vi "Get Property Value.vi"(8 "error in":errorcluster, 10 "Property Type":T1, 11 "Property Type Node":refnum<k20>) -> (0 "error out":errorcluster, 2 "Property Value":variant, 3 "Property Type Node":refnum<k20>)   [LabVIEW 2024, in "Config File Parser.lvlib" / "Property.lvclass"]
uses:
  Property.lvclass
  Property.lvclass/Property.ctl
  <resource>/objmgr/DOMUserDefRef.rc
  <vilib>/xml/NI_XML.lvlib
  Config File Parser.lvlib
  DependentFile.ctl
  <vilib>/xml/Close Reference(Node).vi
  Property Type.ctl
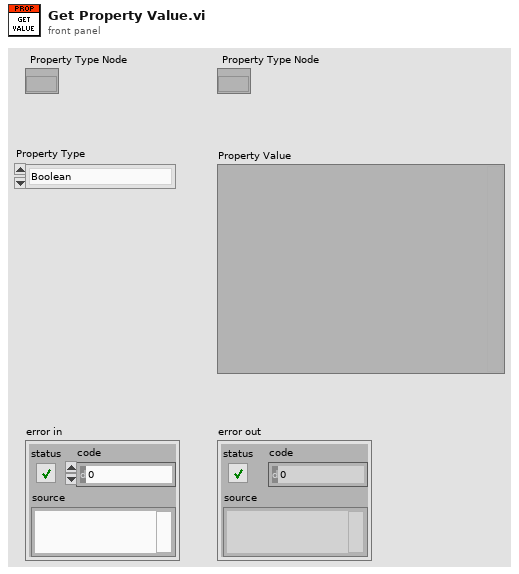
[diagram p1: front panel]
types:
  T1 = typedef "Config File Parser.lvlib/Property.lvclass/Property Type.ctl" = enum16{"Boolean", "Double", "String", "Path", "Dictionary", "DependentFile", "I16", "I32", "I64", "U16", "U32", "U64", "BooleanArray", "DoubleArray", "StringArray", "I16Array", "I32Array", "I64Array", "U16Array", "U32Array", "U64Array"}
  T2 = typedef "Config File Parser.lvlib/Property.lvclass/DependentFile.ctl" = cluster{"Path":string, "Version":string, "RTDestination":string, "ForceDownload":string, "SupportedTarget":string, "MD5":string, " Type":string}
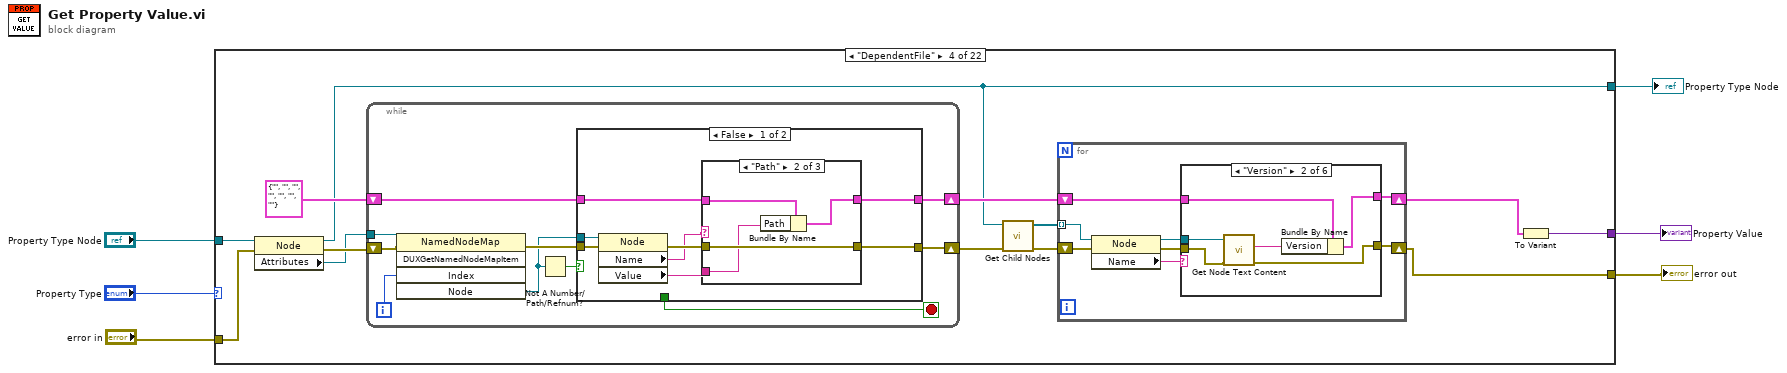
[diagram p0: block diagram]
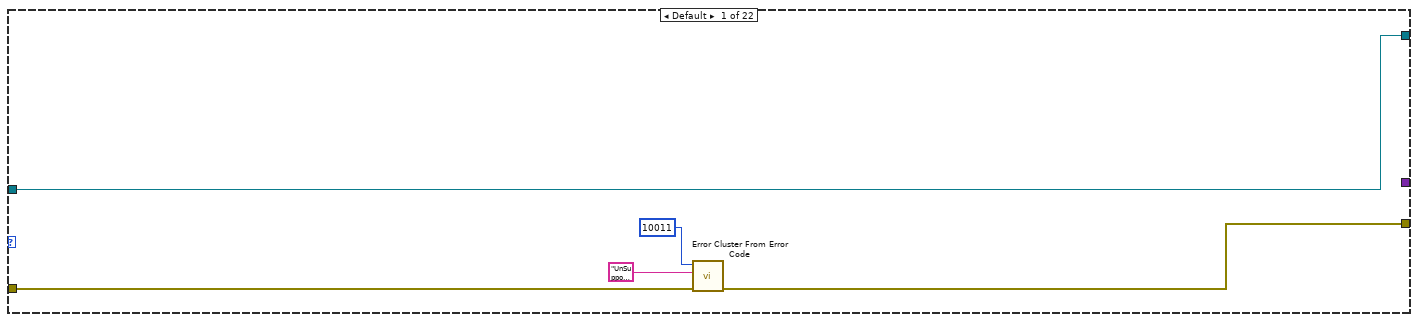
[diagram p2: hidden frame]
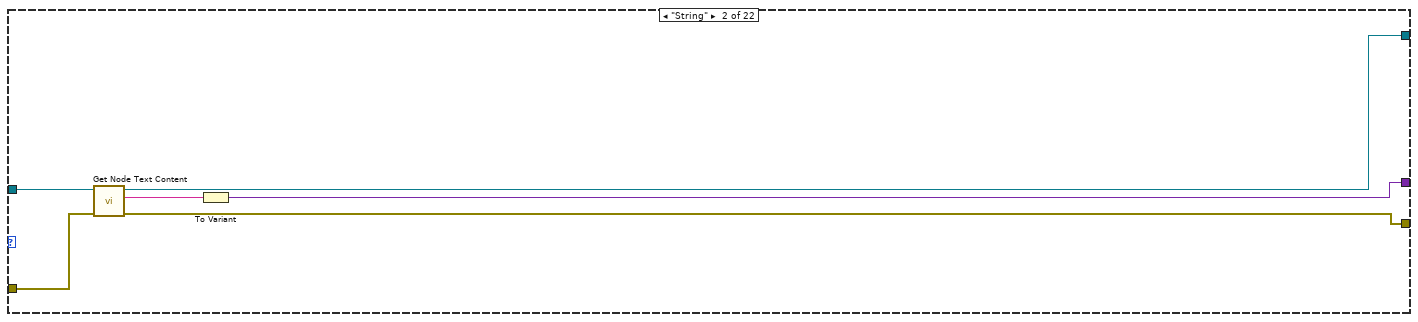
[diagram p3: hidden frame]
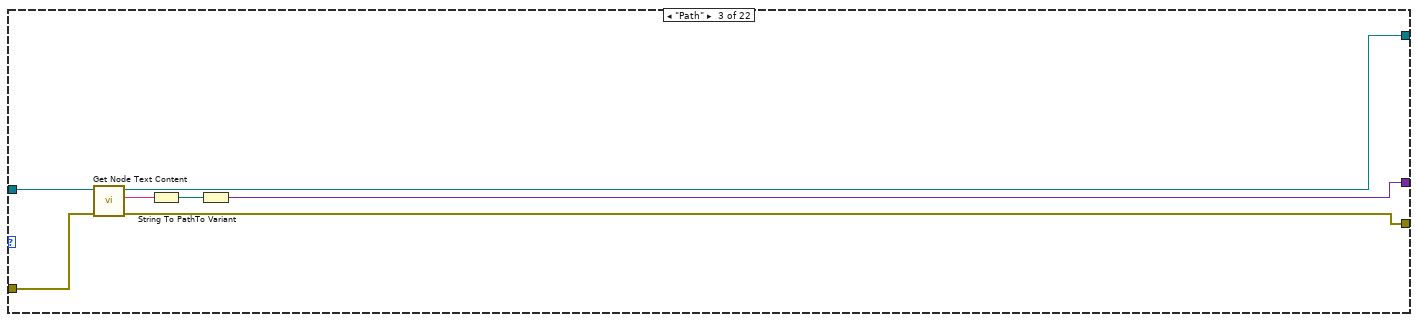
[diagram p4: hidden frame]
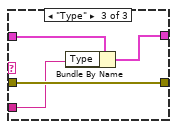
[diagram p6: hidden frame]
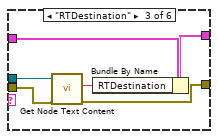
[diagram p9: hidden frame]
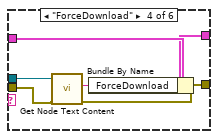
[diagram p10: hidden frame]
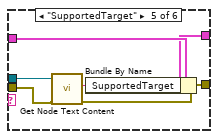
[diagram p11: hidden frame]
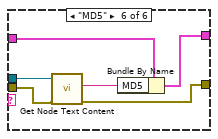
[diagram p12: hidden frame]
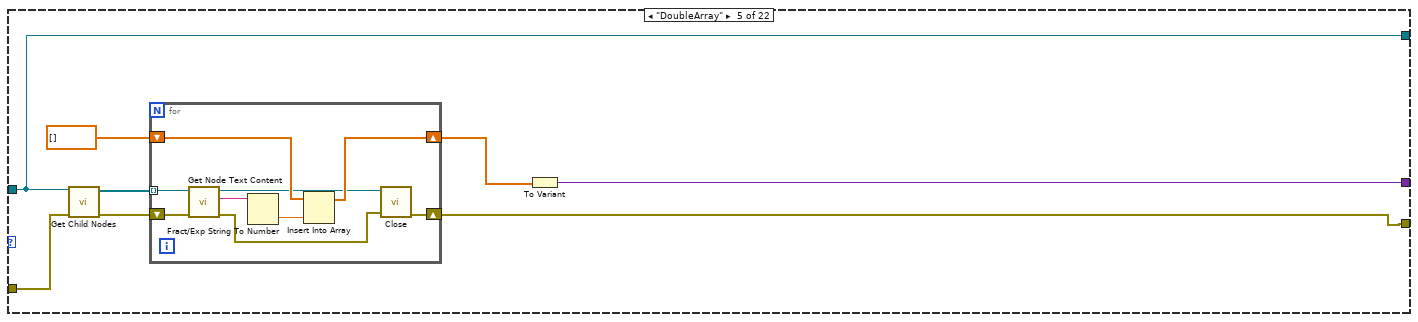
[diagram p13: hidden frame]
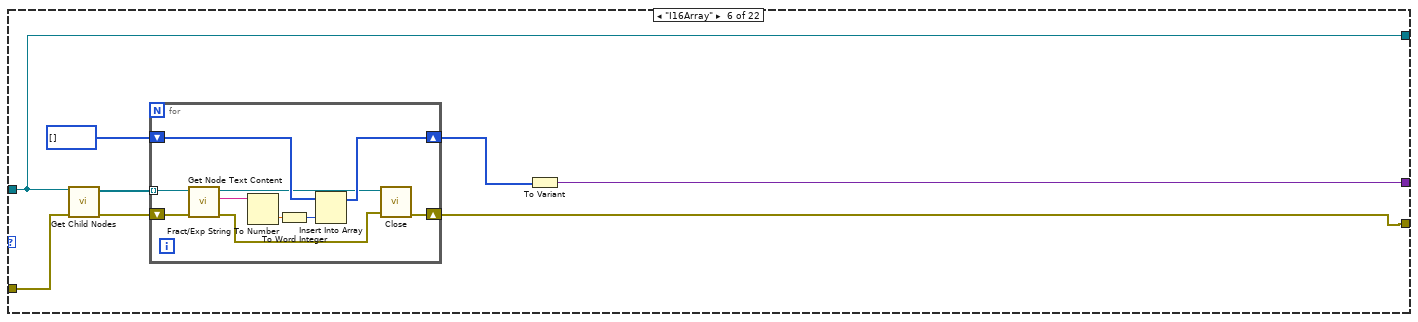
[diagram p14: hidden frame]
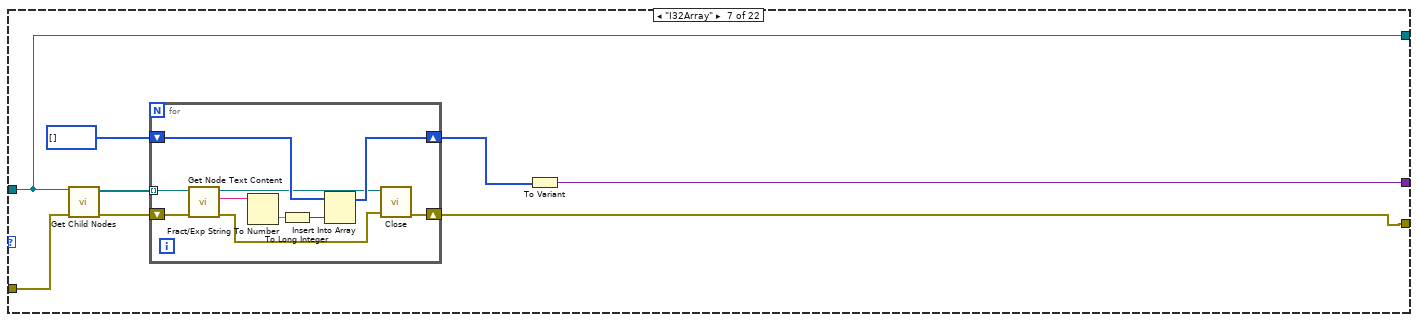
[diagram p15: hidden frame]
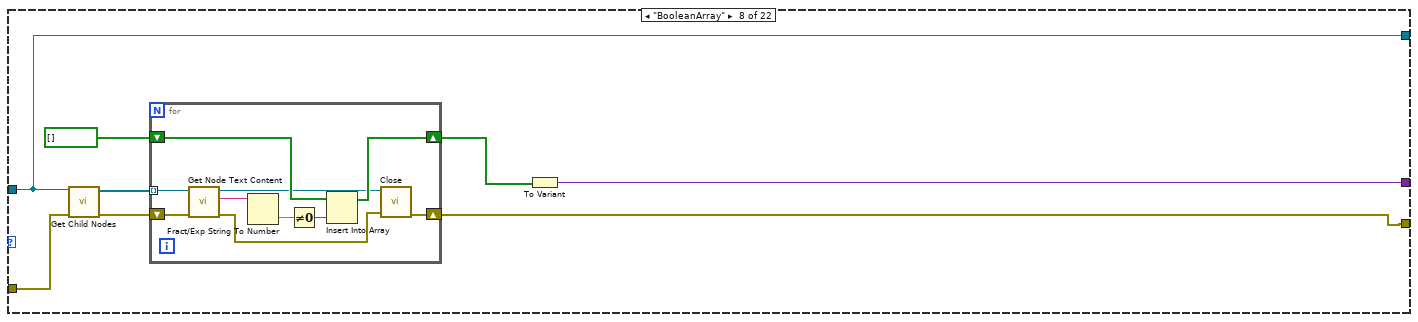
[diagram p16: hidden frame]
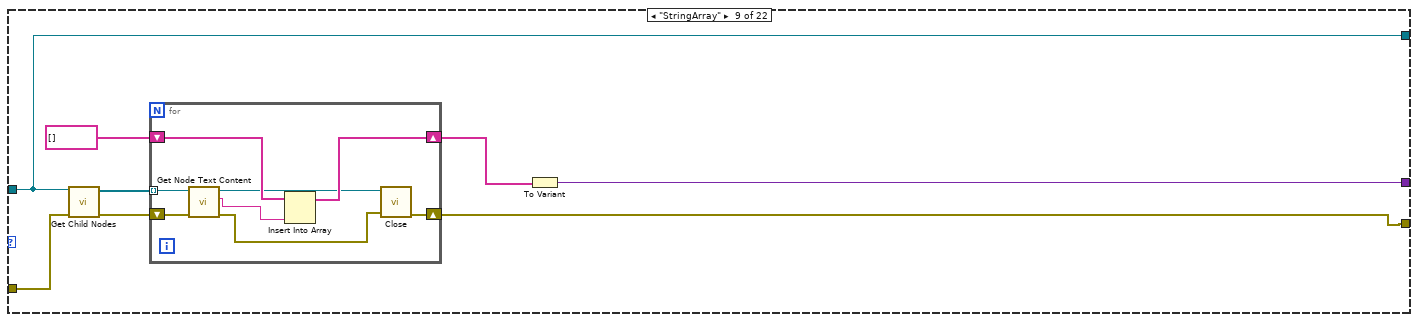
[diagram p17: hidden frame]
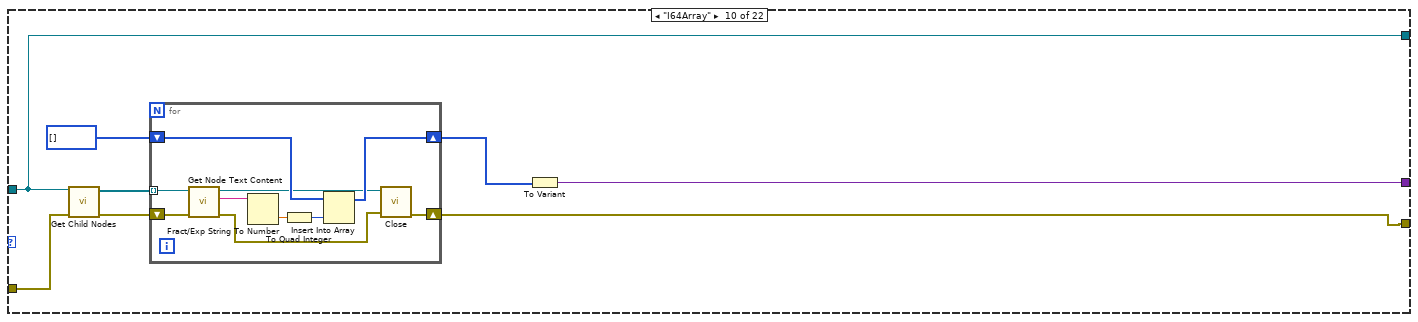
[diagram p18: hidden frame]
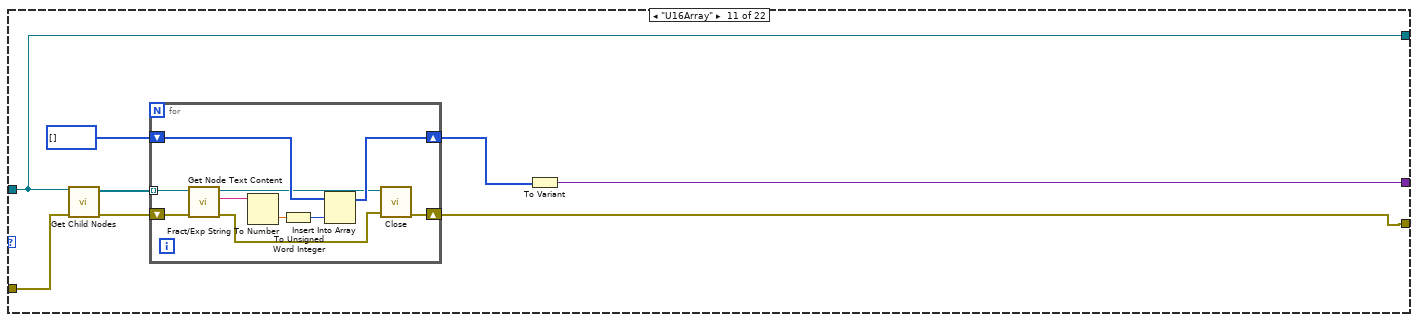
[diagram p19: hidden frame]
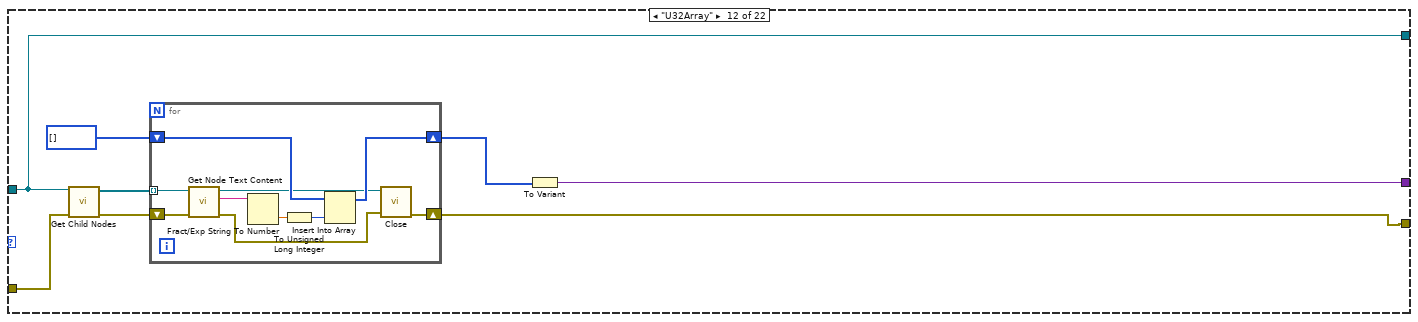
[diagram p20: hidden frame]
diagram:
  n1 = case shown="\"DependentFile\"" "Property Type" {
    tunnel: "Property Type Node" -> [w9 w13 w21 w32 w109 w126 w144 w162 w180 w196 w214 w232 w250 w273 w281 w289 w297 w305 w313 w321 w328 w331]
    tunnel: [_ w15 w22 w30 w111 w128 w146 w164 w182 w198 w216 w234 w252 w268 w276 w284 w292 w300 w308 w318 w325 w333] -> w3
    tunnel: "error in" -> [w11 w17 w24 w37 w115 w132 w150 w168 w186 w202 w220 w238 w256 w275 w283 w291 w299 w307 w315 w323 w330 w338]
    tunnel: [w10 w16 w23 w33 w116 w133 w151 w169 w187 w203 w221 w239 w257 w274 w282 w290 w298 w306 w314 w322 w329 w336] -> w5
    tunnel: [w9 w12 w20 w25 w109 w126 w144 w162 w180 w196 w214 w232 w250 w272 w280 w288 w296 w304 w312 w320 w327 w331] -> w2
    frame Default {
      n2 = call <vilib>:"Error Cluster From Error Code.vi"("error in (no error)"=w11, "error message (\"\")"="UnSupported Property Types are present in the Config File", "error code (0)"=10011) -> ("error out"=w10:errorcluster)  [unwired: 6 in]
    }
    frame "String" {
      n3 = call <vilib>:"Get Node Text Content.vi"("error in (no error)"=w17, "node in"=w13) -> ("error out"=w16:errorcluster, "node text"=w14:string, "node out"=w12:refnum<k20>)  [unwired: 7 in]
      n4 = To Variant(anything=w14) -> (Variant=w15:variant)
    }
    frame "Path" {
      n5 = call <vilib>:"Get Node Text Content.vi"("error in (no error)"=w24, "node in"=w21) -> ("error out"=w23:errorcluster, "node text"=w19:string, "node out"=w20:refnum<k20>)  [unwired: 7 in]
      n6 = String To Path(string=w19) -> (path=w18:path)
      n7 = To Variant(anything=w18) -> (Variant=w22:variant)
    }
    frame "DependentFile" {
      n8 = property class="Node"(reference=w32, error in=w37) -> (reference out=w25:refnum<k20>, error out=w36:errorcluster, "Attributes"=w29:refnum<k20>)
      n9 = while {
        tunnel: w29 -> [w44]
        shift-right: [w45] -> w35
        shift-left: w36 -> [w47]
        shift-right: [w38] -> w27
        shift-left: T2 {"Path"="", "Version"="", "RTDestination"="", "ForceDownload"="", "SupportedTarget"="", "MD5"="", " Type"=""} ("Cluster") -> [w39]
        i -> [w43]
        stop <- w40 stop-if-true
        n10 = invoke class="NamedNodeMap" method="DUXGetNamedNodeMapItem"(reference=w44, error in=w47, "Index"=w43) -> (error out=w46:errorcluster, "Node"=w42:refnum<k20>)  [unwired: 2 in, 3 out]
        n11 = Not A Number/Path/Refnum?(number/path/refnum=w42) -> (NaN/Path/Refnum?=w41:bool)
        n12 = case shown="False" w41 {
          selector: w41 -> [_ w67]
          tunnel: w46 -> [w55 w68]
          tunnel: [w53 w68] -> w45
          tunnel: w42 -> [w52 _]
          tunnel: [_ w67] -> w40
          tunnel: w39 -> [w50 w66]
          tunnel: [w48 w66] -> w38
          frame False {
            n13 = property class="Node"(reference=w52, error in=w55) -> (error out=w54:errorcluster, "Name"=w51:string, "Value"=w49:string)  [unwired: 1 out]
            n14 = case shown="\"Path\"" w51 {
              tunnel: w50 -> [w56 w60 w64]
              tunnel: w49 -> [_ w59 w63]
              tunnel: [w56 w58 w62] -> w48
              tunnel: w54 -> [w57 w61 w65]
              tunnel: [w57 w61 w65] -> w53
              frame "False", Default {
              }
              frame "Path" {
                n15 = Bundle By Name(cluster=w60, "Path"=w59) -> (w58:T2)
              }
              frame "Type" {
                n16 = Bundle By Name(cluster=w64, "Type"=w63) -> (w62:T2)
              }
            }
          }
          frame True {
          }
        }
      }
      n17 = call "Get Child Nodes.vi"("error in"=w35, "Node"=w25) -> ("error out"=w34:errorcluster, "Child Nodes"=w31:refnum<k20>[])  [unwired: 8 in]
      n18 = for {
        tunnel: w31 -> [w73] mode=indexing
        shift-right: [w74] -> w33
        shift-left: w34 -> [w76]
        shift-right: [w69] -> w26
        shift-left: w27 -> [w71]
        n19 = property class="Node"(reference=w73, error in=w76) -> (reference out=w70:refnum<k20>, error out=w75:errorcluster, "Name"=w72:string)
        n20 = case shown="\"Version\"" w72 {
          tunnel: w71 -> [w77 w82 w88 w94 w100 w106]
          tunnel: w70 -> [_ w81 w87 w93 w99 w105]
          tunnel: [w77 w79 w85 w91 w97 w103] -> w69
          tunnel: w75 -> [w78 w84 w90 w96 w102 w108]
          tunnel: [w78 w83 w89 w95 w101 w107] -> w74
          frame "False", Default {
          }
          frame "Version" {
            n21 = call <vilib>:"Get Node Text Content.vi"("error in (no error)"=w84, "node in"=w81) -> ("error out"=w83:errorcluster, "node text"=w80:string)  [unwired: 7 in, 1 out]
            n22 = Bundle By Name(cluster=w82, "Version"=w80) -> (w79:T2)
          }
          frame "RTDestination" {
            n23 = call <vilib>:"Get Node Text Content.vi"("error in (no error)"=w90, "node in"=w87) -> ("error out"=w89:errorcluster, "node text"=w86:string)  [unwired: 7 in, 1 out]
            n24 = Bundle By Name(cluster=w88, "RTDestination"=w86) -> (w85:T2)
          }
          frame "ForceDownload" {
            n25 = call <vilib>:"Get Node Text Content.vi"("error in (no error)"=w96, "node in"=w93) -> ("error out"=w95:errorcluster, "node text"=w92:string)  [unwired: 7 in, 1 out]
            n26 = Bundle By Name(cluster=w94, "ForceDownload"=w92) -> (w91:T2)
          }
          frame "SupportedTarget" {
            n27 = call <vilib>:"Get Node Text Content.vi"("error in (no error)"=w102, "node in"=w99) -> ("error out"=w101:errorcluster, "node text"=w98:string)  [unwired: 7 in, 1 out]
            n28 = Bundle By Name(cluster=w100, "SupportedTarget"=w98) -> (w97:T2)
          }
          frame "MD5" {
            n29 = call <vilib>:"Get Node Text Content.vi"("error in (no error)"=w108, "node in"=w105) -> ("error out"=w107:errorcluster, "node text"=w104:string)  [unwired: 7 in, 1 out]
            n30 = Bundle By Name(cluster=w106, "MD5"=w104) -> (w103:T2)
          }
        }
      }
      n31 = To Variant(anything=w26) -> (Variant=w30:variant)
    }
    frame "DoubleArray" {
      n32 = call "Get Child Nodes.vi"("error in"=w115, "Node"=w109) -> ("error out"=w114:errorcluster, "Child Nodes"=w113:refnum<k20>[])  [unwired: 8 in]
      n33 = for {
        tunnel: w113 -> [w122] mode=indexing
        shift-right: [w118] -> w110
        shift-left: dbl[] [] -> [w119]
        shift-right: [w123] -> w116
        shift-left: w114 -> [w125]
        n34 = call <vilib>:"Get Node Text Content.vi"("error in (no error)"=w125, "node in"=w122) -> ("error out"=w124:errorcluster, "node text"=w121:string, "node out"=w117:refnum<k20>)  [unwired: 7 in]
        n35 = Fract/Exp String To Number(string=w121) -> (number=w120:dbl)  [unwired: 3 in, 1 out]
        n36 = Insert Into Array(array=w119, new element=w120) -> (w118:dbl[])  [unwired: 1 in]
        n37 = call-poly <vilib>:"Close.vi"("error in (no error)"=w124, "node"=w117) -> ("error out"=w123:errorcluster)  [unwired: 7 in]
      }
      n38 = To Variant(anything=w110) -> (Variant=w111:variant)
    }
    frame "I16Array" {
      n39 = call "Get Child Nodes.vi"("error in"=w132, "Node"=w126) -> ("error out"=w131:errorcluster, "Child Nodes"=w130:refnum<k20>[])  [unwired: 8 in]
      n40 = for {
        tunnel: w130 -> [w140] mode=indexing
        shift-right: [w136] -> w127
        shift-left: i16[] [] -> [w137]
        shift-right: [w141] -> w133
        shift-left: w131 -> [w143]
        n41 = call <vilib>:"Get Node Text Content.vi"("error in (no error)"=w143, "node in"=w140) -> ("error out"=w142:errorcluster, "node text"=w139:string, "node out"=w135:refnum<k20>)  [unwired: 7 in]
        n42 = Fract/Exp String To Number(string=w139) -> (number=w138:dbl)  [unwired: 3 in, 1 out]
        n43 = To Word Integer(number=w138) -> (16bit integer=w134:i16)
        n44 = Insert Into Array(array=w137, new element=w134) -> (w136:i16[])  [unwired: 1 in]
        n45 = call-poly <vilib>:"Close.vi"("error in (no error)"=w142, "node"=w135) -> ("error out"=w141:errorcluster)  [unwired: 7 in]
      }
      n46 = To Variant(anything=w127) -> (Variant=w128:variant)
    }
    frame "I32Array" {
      n47 = call "Get Child Nodes.vi"("error in"=w150, "Node"=w144) -> ("error out"=w149:errorcluster, "Child Nodes"=w148:refnum<k20>[])  [unwired: 8 in]
      n48 = for {
        tunnel: w148 -> [w158] mode=indexing
        shift-right: [w154] -> w145
        shift-left: i32[] [] -> [w155]
        shift-right: [w159] -> w151
        shift-left: w149 -> [w161]
        n49 = call <vilib>:"Get Node Text Content.vi"("error in (no error)"=w161, "node in"=w158) -> ("error out"=w160:errorcluster, "node text"=w157:string, "node out"=w153:refnum<k20>)  [unwired: 7 in]
        n50 = Fract/Exp String To Number(string=w157) -> (number=w156:dbl)  [unwired: 3 in, 1 out]
        n51 = To Long Integer(number=w156) -> (32bit integer=w152:i32)
        n52 = Insert Into Array(array=w155, new element=w152) -> (w154:i32[])  [unwired: 1 in]
        n53 = call-poly <vilib>:"Close.vi"("error in (no error)"=w160, "node"=w153) -> ("error out"=w159:errorcluster)  [unwired: 7 in]
      }
      n54 = To Variant(anything=w145) -> (Variant=w146:variant)
    }
    frame "BooleanArray" {
      n55 = call "Get Child Nodes.vi"("error in"=w168, "Node"=w162) -> ("error out"=w167:errorcluster, "Child Nodes"=w166:refnum<k20>[])  [unwired: 8 in]
      n56 = for {
        tunnel: w166 -> [w176] mode=indexing
        shift-right: [w172] -> w163
        shift-left: bool[] [] -> [w173]
        shift-right: [w177] -> w169
        shift-left: w167 -> [w179]
        n57 = call <vilib>:"Get Node Text Content.vi"("error in (no error)"=w179, "node in"=w176) -> ("error out"=w178:errorcluster, "node text"=w175:string, "node out"=w171:refnum<k20>)  [unwired: 7 in]
        n58 = Fract/Exp String To Number(string=w175) -> (number=w174:dbl)  [unwired: 3 in, 1 out]
        n59 = Not Equal To 0?(x=w174) -> (x != 0?=w170:bool)
        n60 = Insert Into Array(array=w173, new element=w170) -> (w172:bool[])  [unwired: 1 in]
        n61 = call-poly <vilib>:"Close.vi"("error in (no error)"=w178, "node"=w171) -> ("error out"=w177:errorcluster)  [unwired: 7 in]
      }
      n62 = To Variant(anything=w163) -> (Variant=w164:variant)
    }
    frame "StringArray" {
      n63 = call "Get Child Nodes.vi"("error in"=w186, "Node"=w180) -> ("error out"=w185:errorcluster, "Child Nodes"=w184:refnum<k20>[])  [unwired: 8 in]
      n64 = for {
        tunnel: w184 -> [w192] mode=indexing
        shift-right: [w190] -> w181
        shift-left: string[] [] -> [w191]
        shift-right: [w193] -> w187
        shift-left: w185 -> [w195]
        n65 = call <vilib>:"Get Node Text Content.vi"("error in (no error)"=w195, "node in"=w192) -> ("error out"=w194:errorcluster, "node text"=w188:string, "node out"=w189:refnum<k20>)  [unwired: 7 in]
        n66 = Insert Into Array(array=w191, new element=w188) -> (w190:string[])  [unwired: 1 in]
        n67 = call-poly <vilib>:"Close.vi"("error in (no error)"=w194, "node"=w189) -> ("error out"=w193:errorcluster)  [unwired: 7 in]
      }
      n68 = To Variant(anything=w181) -> (Variant=w182:variant)
    }
    frame "I64Array" {
      n69 = call "Get Child Nodes.vi"("error in"=w202, "Node"=w196) -> ("error out"=w201:errorcluster, "Child Nodes"=w200:refnum<k20>[])  [unwired: 8 in]
      n70 = for {
        tunnel: w200 -> [w210] mode=indexing
        shift-right: [w206] -> w197
        shift-left: i64[] [] -> [w207]
        shift-right: [w211] -> w203
        shift-left: w201 -> [w213]
        n71 = call <vilib>:"Get Node Text Content.vi"("error in (no error)"=w213, "node in"=w210) -> ("error out"=w212:errorcluster, "node text"=w209:string, "node out"=w205:refnum<k20>)  [unwired: 7 in]
        n72 = Fract/Exp String To Number(string=w209) -> (number=w208:dbl)  [unwired: 3 in, 1 out]
        n73 = To Quad Integer(1:w208) -> (0:w204:i64)
        n74 = Insert Into Array(array=w207, new element=w204) -> (w206:i64[])  [unwired: 1 in]
        n75 = call-poly <vilib>:"Close.vi"("error in (no error)"=w212, "node"=w205) -> ("error out"=w211:errorcluster)  [unwired: 7 in]
      }
      n76 = To Variant(anything=w197) -> (Variant=w198:variant)
    }
    frame "U16Array" {
      n77 = call "Get Child Nodes.vi"("error in"=w220, "Node"=w214) -> ("error out"=w219:errorcluster, "Child Nodes"=w218:refnum<k20>[])  [unwired: 8 in]
      n78 = for {
        tunnel: w218 -> [w228] mode=indexing
        shift-right: [w224] -> w215
        shift-left: u16[] [] -> [w225]
        shift-right: [w229] -> w221
        shift-left: w219 -> [w231]
        n79 = call <vilib>:"Get Node Text Content.vi"("error in (no error)"=w231, "node in"=w228) -> ("error out"=w230:errorcluster, "node text"=w227:string, "node out"=w223:refnum<k20>)  [unwired: 7 in]
        n80 = Fract/Exp String To Number(string=w227) -> (number=w226:dbl)  [unwired: 3 in, 1 out]
        n81 = To Unsigned Word Integer(number=w226) -> (unsigned 16bit integer=w222:u16)
        n82 = Insert Into Array(array=w225, new element=w222) -> (w224:u16[])  [unwired: 1 in]
        n83 = call-poly <vilib>:"Close.vi"("error in (no error)"=w230, "node"=w223) -> ("error out"=w229:errorcluster)  [unwired: 7 in]
      }
      n84 = To Variant(anything=w215) -> (Variant=w216:variant)
    }
    frame "U32Array" {
      n85 = call "Get Child Nodes.vi"("error in"=w238, "Node"=w232) -> ("error out"=w237:errorcluster, "Child Nodes"=w236:refnum<k20>[])  [unwired: 8 in]
      n86 = for {
        tunnel: w236 -> [w246] mode=indexing
        shift-right: [w242] -> w233
        shift-left: u32[] [] -> [w243]
        shift-right: [w247] -> w239
        shift-left: w237 -> [w249]
        n87 = call <vilib>:"Get Node Text Content.vi"("error in (no error)"=w249, "node in"=w246) -> ("error out"=w248:errorcluster, "node text"=w245:string, "node out"=w241:refnum<k20>)  [unwired: 7 in]
        n88 = Fract/Exp String To Number(string=w245) -> (number=w244:dbl)  [unwired: 3 in, 1 out]
        n89 = To Unsigned Long Integer(number=w244) -> (unsigned 32bit integer=w240:u32)
        n90 = Insert Into Array(array=w243, new element=w240) -> (w242:u32[])  [unwired: 1 in]
        n91 = call-poly <vilib>:"Close.vi"("error in (no error)"=w248, "node"=w241) -> ("error out"=w247:errorcluster)  [unwired: 7 in]
      }
      n92 = To Variant(anything=w233) -> (Variant=w234:variant)
    }
    frame "U64Array" {
      n93 = call "Get Child Nodes.vi"("error in"=w256, "Node"=w250) -> ("error out"=w255:errorcluster, "Child Nodes"=w254:refnum<k20>[])  [unwired: 8 in]
      n94 = for {
        tunnel: w254 -> [w264] mode=indexing
        shift-right: [w260] -> w251
        shift-left: u64[] [] -> [w261]
        shift-right: [w265] -> w257
        shift-left: w255 -> [w267]
        n95 = call <vilib>:"Get Node Text Content.vi"("error in (no error)"=w267, "node in"=w264) -> ("error out"=w266:errorcluster, "node text"=w263:string, "node out"=w259:refnum<k20>)  [unwired: 7 in]
        n96 = Fract/Exp String To Number(string=w263) -> (number=w262:dbl)  [unwired: 3 in, 1 out]
        n97 = To Unsigned Quad Integer(1:w262) -> (0:w258:u64)
        n98 = Insert Into Array(array=w261, new element=w258) -> (w260:u64[])  [unwired: 1 in]
        n99 = call-poly <vilib>:"Close.vi"("error in (no error)"=w266, "node"=w259) -> ("error out"=w265:errorcluster)  [unwired: 7 in]
      }
      n100 = To Variant(anything=w251) -> (Variant=w252:variant)
    }
    frame "U32" {
      n101 = call <vilib>:"Get Node Text Content.vi"("error in (no error)"=w275, "node in"=w273) -> ("error out"=w274:errorcluster, "node text"=w271:string, "node out"=w272:refnum<k20>)  [unwired: 7 in]
      n102 = Fract/Exp String To Number(string=w271) -> (number=w270:dbl)  [unwired: 3 in, 1 out]
      n103 = To Unsigned Long Integer(number=w270) -> (unsigned 32bit integer=w269:u32)
      n104 = To Variant(anything=w269) -> (Variant=w268:variant)
    }
    frame "U16" {
      n105 = call <vilib>:"Get Node Text Content.vi"("error in (no error)"=w283, "node in"=w281) -> ("error out"=w282:errorcluster, "node text"=w279:string, "node out"=w280:refnum<k20>)  [unwired: 7 in]
      n106 = Fract/Exp String To Number(string=w279) -> (number=w278:dbl)  [unwired: 3 in, 1 out]
      n107 = To Unsigned Word Integer(number=w278) -> (unsigned 16bit integer=w277:u16)
      n108 = To Variant(anything=w277) -> (Variant=w276:variant)
    }
    frame "U64" {
      n109 = call <vilib>:"Get Node Text Content.vi"("error in (no error)"=w291, "node in"=w289) -> ("error out"=w290:errorcluster, "node text"=w287:string, "node out"=w288:refnum<k20>)  [unwired: 7 in]
      n110 = Fract/Exp String To Number(string=w287) -> (number=w286:dbl)  [unwired: 3 in, 1 out]
      n111 = To Unsigned Quad Integer(1:w286) -> (0:w285:u64)
      n112 = To Variant(anything=w285) -> (Variant=w284:variant)
    }
    frame "I16" {
      n113 = call <vilib>:"Get Node Text Content.vi"("error in (no error)"=w299, "node in"=w297) -> ("error out"=w298:errorcluster, "node text"=w295:string, "node out"=w296:refnum<k20>)  [unwired: 7 in]
      n114 = Fract/Exp String To Number(string=w295) -> (number=w294:dbl)  [unwired: 3 in, 1 out]
      n115 = To Word Integer(number=w294) -> (16bit integer=w293:i16)
      n116 = To Variant(anything=w293) -> (Variant=w292:variant)
    }
    frame "I32" {
      n117 = call <vilib>:"Get Node Text Content.vi"("error in (no error)"=w307, "node in"=w305) -> ("error out"=w306:errorcluster, "node text"=w303:string, "node out"=w304:refnum<k20>)  [unwired: 7 in]
      n118 = Fract/Exp String To Number(string=w303) -> (number=w302:dbl)  [unwired: 3 in, 1 out]
      n119 = To Long Integer(number=w302) -> (32bit integer=w301:i32)
      n120 = To Variant(anything=w301) -> (Variant=w300:variant)
    }
    frame "I64" {
      n121 = call <vilib>:"Get Node Text Content.vi"("error in (no error)"=w315, "node in"=w313) -> ("error out"=w314:errorcluster, "node text"=w311:string, "node out"=w312:refnum<k20>)  [unwired: 7 in]
      n122 = Fract/Exp String To Number(string=w311) -> (number=w310:dbl)  [unwired: 3 in, 1 out]
      n123 = To Quad Integer(1:w310) -> (0:w309:i64)
      n124 = To Variant(anything=w309) -> (Variant=w308:variant)
    }
    frame "Boolean" {
      n125 = call <vilib>:"Get Node Text Content.vi"("error in (no error)"=w323, "node in"=w321) -> ("error out"=w322:errorcluster, "node text"=w319:string, "node out"=w320:refnum<k20>)  [unwired: 7 in]
      n126 = Fract/Exp String To Number(string=w319) -> (number=w316:dbl)  [unwired: 3 in, 1 out]
      n127 = Not Equal To 0?(x=w316) -> (x != 0?=w317:bool)
      n128 = To Variant(anything=w317) -> (Variant=w318:variant)
    }
    frame "Double" {
      n129 = call <vilib>:"Get Node Text Content.vi"("error in (no error)"=w330, "node in"=w328) -> ("error out"=w329:errorcluster, "node text"=w326:string, "node out"=w327:refnum<k20>)  [unwired: 7 in]
      n130 = Fract/Exp String To Number(string=w326) -> (number=w324:dbl)  [unwired: 3 in, 1 out]
      n131 = To Variant(anything=w324) -> (Variant=w325:variant)
    }
    frame "Dictionary" {
      w335 = map{string, dbl} {}  # Size: 0
      n132 = call "Get Child Nodes.vi"("error in"=w338, "Node"=w331) -> ("error out"=w337:errorcluster, "Child Nodes"=w334:refnum<k20>[])  [unwired: 8 in]
      n133 = for {
        shift-right: [w344] -> w332
        shift-left: w335 -> [w345]
        tunnel: w334 -> [w343] mode=indexing
        shift-right: [w347] -> w336
        shift-left: w337 -> [w350]
        n134 = property class="Node"(reference=w343, error in=w350) -> (reference out=w339:refnum<k20>, error out=w351:errorcluster, "Attributes"=w346:refnum<k20>)
        n135 = invoke class="NamedNodeMap" method="DUXGetNamedItem"(reference=w346, error in=w351, "Name"="Key") -> (error out=w349:errorcluster, "Node"=w341:refnum<k20>)  [unwired: 2 in, 3 out]
        n136 = Not A Number/Path/Refnum?(number/path/refnum=w341) -> (NaN/Path/Refnum?=w340:bool)
        n137 = case shown="False" w340 {
          tunnel: w341 -> [w359 _]
          tunnel: w339 -> [w358 _]
          tunnel: w345 -> [w356 w380]
          tunnel: [w355 w380] -> w344
          tunnel: w349 -> [w363 w384]
          tunnel: [w360 w383] -> w348
          frame False {
            n138 = call <vilib>:"Get Node Text Content.vi"("error in (no error)"=w363, "node in"=w359) -> ("error out"=w362:errorcluster, "node text"=w357:string, "node out"=w353:refnum<k20>)  [unwired: 7 in]
            n139 = call <vilib>:"Get First Non-Text Child.vi"("error in (no error)"=w362, "node in"=w358) -> ("error out"=w364:errorcluster, "found child node?"=w352:bool, "child node"=w354:refnum<k20>)  [unwired: 6 in, 1 out]
            n140 = case shown="True" w352 {
              tunnel: w364 -> [w369 w379]
              tunnel: w357 -> [_ w375]
              tunnel: w356 -> [w365 w373]
              tunnel: [w365 w372] -> w355
              tunnel: w354 -> [_ w371]
              tunnel: [w368 w377] -> w361
              frame False {
                n141 = call <vilib>:"Error Cluster From Error Code.vi"("error in (no error)"=w369, "error message (\"\")"="A value is missing for one or more keys in the dictionary-typed property", "error code (0)"=10017) -> ("error out"=w368:errorcluster)  [unwired: 6 in]
              }
              frame True {
                n142 = call <vilib>:"Get Node Text Content.vi"("error in (no error)"=w379, "node in"=w371) -> ("error out"=w378:errorcluster, "node text"=w376:string, "node out"=w370:refnum<k20>)  [unwired: 7 in]
                n143 = Fract/Exp String To Number(string=w376) -> (number=w374:dbl)  [unwired: 3 in, 1 out]
                n144 = Insert Into Map(map in=w373, key=w375, value=w374) -> (map out=w372:map{string, dbl})  [unwired: 2 out]
                n145 = call-poly <vilib>:"Close.vi"("error in (no error)"=w378, "node"=w370) -> ("error out"=w377:errorcluster)  [unwired: 7 in]
              }
            }
            n146 = call-poly <vilib>:"Close.vi"("error in (no error)"=w361, "node"=w353) -> ("error out"=w360:errorcluster)  [unwired: 7 in]
          }
          frame True {
            n147 = call <vilib>:"Error Cluster From Error Code.vi"("error in (no error)"=w384, "error message (\"\")"="Key does not exist for the Dictionary Typed Property", "error code (0)"=10016) -> ("error out"=w383:errorcluster)  [unwired: 6 in]
          }
        }
        n148 = call-poly <vilib>:"Close.vi"("error in (no error)"=w348, "node"=w339) -> ("error out"=w347:errorcluster)  [unwired: 7 in]
      }
      n149 = To Variant(anything=w332) -> (Variant=w333:variant)
    }
  }
  "Property Value" <- w3
  "error out" <- w5
  "Property Type Node" <- w2
